vi "Store Configuration Parameters.vi"(8 "error in (no error)":errorcluster, 10 "refnum":T1, 11 "HW Configuration in":refnum<class "HW Configuration.lvclass">) -> (0 "error out":errorcluster, 2 "refnum out":T1, 3 "HW Configuration out":refnum<class "HW Configuration.lvclass">)   [LabVIEW 2017, in "Hardware.lvlib" / "HW Configuration.lvclass"]
uses:
  HW Configuration.lvclass
  C:/Program Files (x86)/National Instruments/LabVIEW 2017/user.lib/Configuration Dialog Actor/Configuration.lvclass
  <vilib>/Utility/config.llb/Config Data RefNum.ctl
  <userlib>/Configuration Dialog Actor/Configuration.lvclass/Configuration.ctl
  HW Configuration.lvclass/HW Configuration.ctl
  <userlib>/Configuration Dialog Actor/Configuration.lvclass
  <vilib>/Utility/config.llb/NI_LVConfig.lvlib
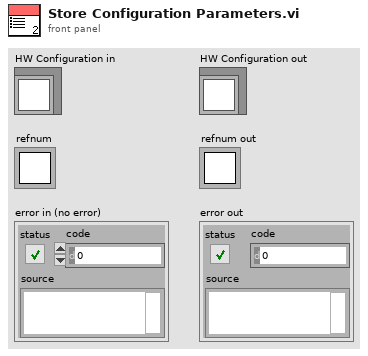
[diagram p1: front panel]
types:
  T1 = typedef "NI_LVConfig.lvlib/Config Data RefNum.ctl" = refnum<k1>
  T2 = cluster{"Device Name":string, "Channel Mapping (Device -> Channel)":string[][]}
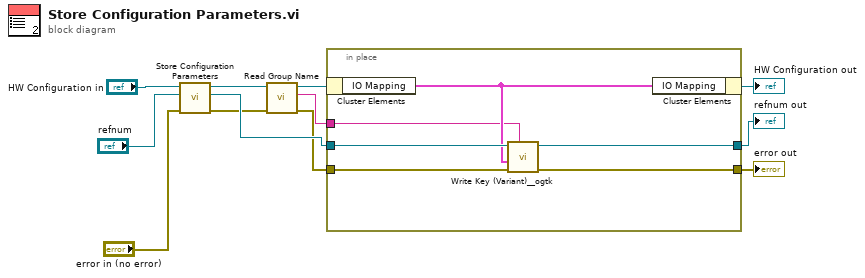
[diagram p0: block diagram]
diagram:
  n1 = call-parent "Store Configuration Parameters.vi"("error in (no error)"="error in (no error)", "refnum"="refnum", "Configuration in"="HW Configuration in") -> ("error out"=w5:errorcluster, "refnum out"=w8:T1, "Configuration out"=w12:refnum<class "HW Configuration.lvclass">)  [unwired: 6 in]
  n2 = call <userlib>:"Read Group Name.vi"("error in (no error)"=w5, "Configuration in"=w12) -> ("error out"=w4:errorcluster, "Group Name"=w6:string, "Configuration out"=w7:refnum<class "HW Configuration.lvclass">)  [unwired: 7 in]
  n3 = in-place {
    in-place-border: w8 -> [w18]
    in-place-border: [w17] -> w3
    in-place-border: [w16] -> w1
    in-place-border: w4 -> [w14]
    in-place-border: w6 -> [w13]
    n4 = in-place-cluster #1(w7) -> ("IO Mapping"=w15:T2)
    n5 = call <userlib>:"Write Key (Variant)__ogtk.vi"("section"=w13, "error in (no error)"=w14, "key-value"=w15, "refnum"=w18) -> ("error out"=w16:errorcluster, "refnum out"=w17:T1)  [unwired: 6 in]
    n6 = in-place-cluster #1("IO Mapping"=w15) -> (→"HW Configuration out":refnum<class "HW Configuration.lvclass">)
  }
  "error out" <- w1
  "refnum out" <- w3
